vi "Move Temp pdf to Folder_ABB.vi"(7 "Month Folder":path, 8 "error in (no error)":errorcluster, 11 "Report  path":path) -> ()   [LabVIEW 2017]
uses:
  ABB global.vi
panel:
  out "Current test":path
  out "Temp report folder":path=path "C:/Program Files/National Instruments/LabVIEW 7.1/LabView 7.1 Apps/ABB motor test/report templates"
  out "String":string="Waiting for PDF....."
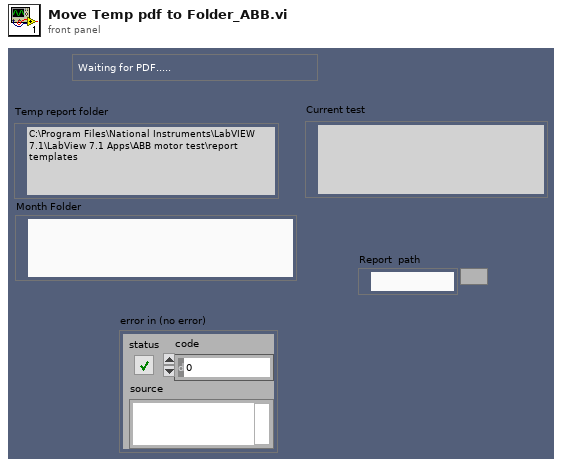
[diagram p1: front panel]
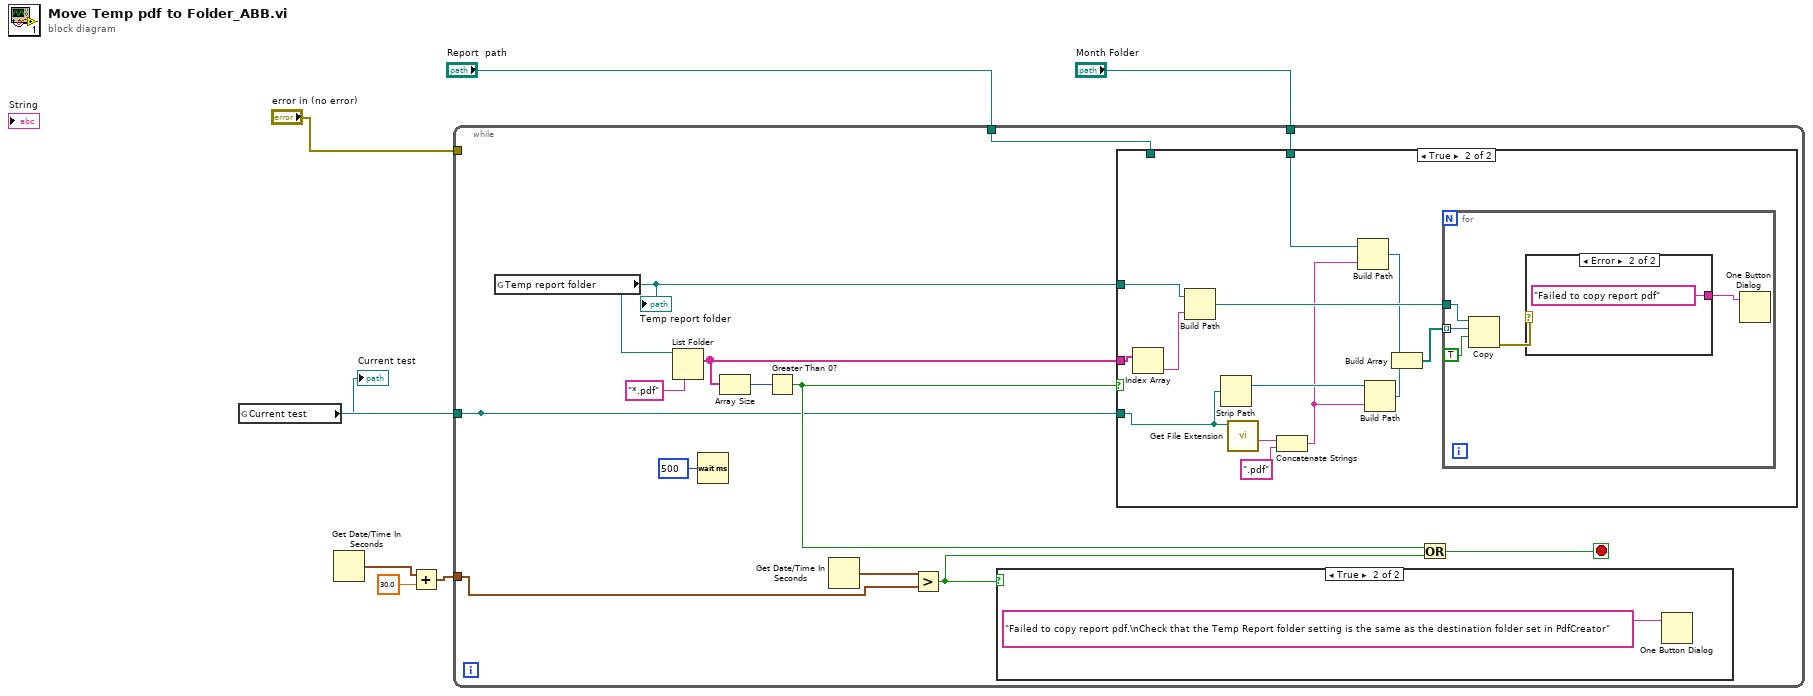
[diagram p0: block diagram]
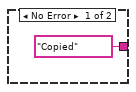
[diagram p4: hidden frame]
diagram:
  n1 = global read "ABB global.vi" "Current test"() -> (w3:path)
  n2 = Get Date/Time In Seconds() -> (seconds since 1Jan1904=w6:timestamp)
  n3 = Add(x=w6, y=30.0) -> (x+y=w4:timestamp)
  n4 = while {
    tunnel: "error in (no error)" -> [_]
    tunnel: "Report  path" -> [w16]
    tunnel: w4 -> [w11]
    tunnel: w3 -> [w13]
    tunnel: [w13] -> w2
    tunnel: "Month Folder" -> [w9]
    stop <- w15 stop-if-true
    n5 = global read "ABB global.vi" "Temp report folder"() -> (w18:path)
    "Temp report folder" <- w18
    n6 = List Folder(path=w18, pattern="*.pdf") -> (filenames=w17:string[])  [unwired: 2 in, 3 out]
    n7 = Wait (ms)(milliseconds to wait=u32 500) -> ()  [unwired: 1 out]
    n8 = Array Size(array=w17) -> (size(s)=w19:i32)
    n9 = Greater Than 0?(x=w19) -> (x > 0?=w14:bool)
    n10 = Get Date/Time In Seconds() -> (seconds since 1Jan1904=w12:timestamp)
    n11 = Greater?(x=w12, y=w11) -> (0:w10:bool)
    n12 = case shown="True" w10 {
      frame False {
      }
      frame True {
        n13 = One Button Dialog(message="Failed to copy report pdf.\nCheck that the Temp Report folder setting is the same as the destination folder set in PdfCreator") -> ()  [unwired: 1 in, 1 out]
      }
    }
    n14 = case shown="True" w14 {
      tunnel: w18 -> [_ w35]
      tunnel: w17 -> [_ w34]
      tunnel: w16 -> [_ _]
      tunnel: w13 -> [_ w29]
      tunnel: w9 -> [_ w25]
      frame False {
      }
      frame True {
        n15 = Index Array(array=w34) -> (element=w33:string)  [unwired: 1 in]
        n16 = Build Path(base path=w35, name or relative path=w33) -> (appended path=w32:path)
        n17 = Strip Path(path=w29) -> (stripped path=w28:path)  [unwired: 1 out]
        n18 = call <vilib>:"Get File Extension.vi"("file"=w29) -> ("filename without extension"=w31:string)  [unwired: 6 in, 4 out]
        n19 = Concatenate Strings(w31, ".pdf" ("string")) -> (w26:string)
        n20 = Build Path(base path=w25, name or relative path=w26) -> (appended path=w24:path)
        n21 = Build Path(base path=w28, name or relative path=w26) -> (appended path=w27:path)
        n22 = Build Array(w24, w27) -> (w23:path[])
        n23 = for {
          tunnel: w32 -> [w40]
          tunnel: w23 -> [w36] mode=indexing
          n24 = Copy(9:TRUE ("overwrite (F)"), 10:w36, 11:w40) -> (0:w39:errorcluster)  [unwired: 2 in, 2 out]
          n25 = case shown="Error" w39 {
            tunnel: ["Copied" "Failed to copy report pdf"] -> w38
            frame No Error {
            }
            frame Error {
            }
          }
          n26 = One Button Dialog(message=w38) -> ()  [unwired: 1 in, 1 out]
        }
      }
    }
    n27 = Or(x=w14, y=w10) -> (x .or. y?=w15:bool)
  }
  "Current test" <- w2
